vi "http XML send receive.vi"(4 "error in (no error)":errorcluster, 5 "IP-Adresse (localhost)":string="127.0.0.1", 7 "XML Request":string) -> (0 "error out":errorcluster, 2 "Response Body (XML)":string, 3 "Response Header":string)   [LabVIEW 2020, in "FT-IR.lvlib" / "TOOLweb Interface.lvlib" / "TOOLweb Interface Hilfs-VIs.lvlib"]
doc: "Der als XML-Text-Message übergebene\"XML Request\" wird mit http-POST-Header an die Anwendung ToolWeb/Cmd auf dem Rechner mit der übergebenen IP-Adresse (unverbunden: localhost) gesendet. Das Protokoll ist HTTP 1.1 auf TCP/IP.\nDie Antwort von TOOLweb wird in Response Header (bis Content-Length) und Response Body (XML) aufgeteilt. \"Response Body\" ist direkt als XML-Message auswertbar."
uses:
  TOOLweb Interface Hilfs-VIs.lvlib
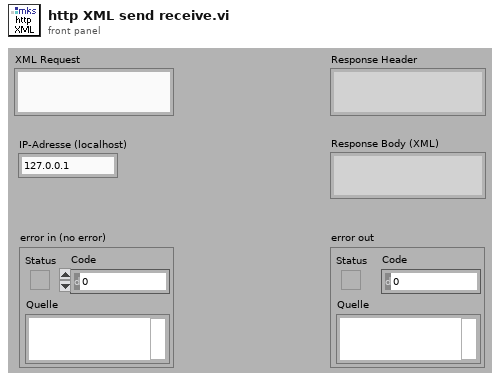
[diagram p1: front panel]
types:
  T1 = enum16{"Standard", "Buffered", "CRLF", "Immediate"}
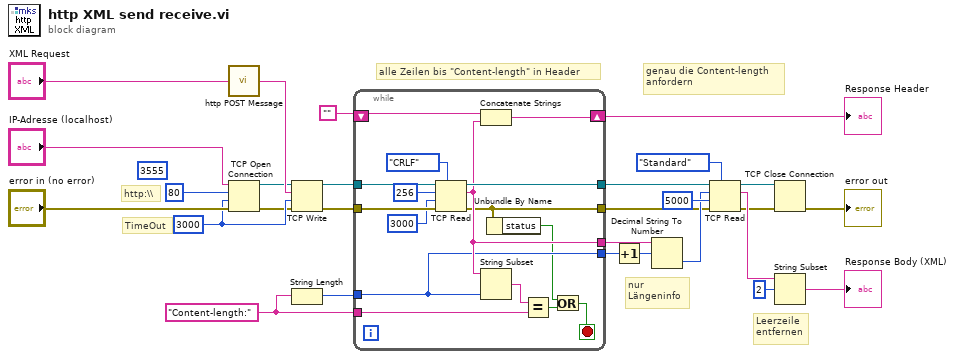
[diagram p0: block diagram]
diagram:
  (unwired) u16 3555 ("Netzwerk-Port oder -Dienst")
  w26 = "Content-length:"
  w7 = 3000 ("Timeout in ms (60000)")
  # "genau die Content-length\nanfordern"
  # "alle Zeilen bis \"Content-length\" in Header"
  # "Leerzeile\nentfernen"
  # "nur\nLängeninfo"
  # "TimeOut"
  # "http:\\\\"
  n1 = call "http POST Message.vi"("http Message Body"="XML Request") -> ("http POST Message"=w24:string)
  n2 = TCP Open Connection(address="IP-Adresse (localhost)", remote port or service name=u16 80 ("Netzwerk-Port oder -Dienst"), timeout ms (60000)=w7, error in (no error)="error in (no error)") -> (connection ID=w4:refnum<k5>, error out=w3:errorcluster)  [unwired: 1 out]
  n3 = TCP Write(connection ID=w4, data in=w24, error in (no error)=w3, 9:w7) -> (connection ID out=w5:refnum<k5>, error out=w6:errorcluster)  [unwired: 1 out]
  n4 = String Length(string=w26) -> (length=w25:i32)
  n5 = while {
    tunnel: w5 -> [w44]
    tunnel: w6 -> [w43]
    tunnel: [w32] -> w8
    tunnel: [w39] -> w10
    shift-right: [w37] -> w14
    shift-left: "" -> [w38]
    tunnel: [w35] -> w15
    tunnel: w25 -> [w33]
    tunnel: w26 -> [w34]
    tunnel: [w33] -> w28
    stop <- w29 stop-if-true
    n6 = TCP Read(connection ID=w44, bytes to read=256 ("Zu lesende Bytes"), error in (no error)=w43, 7:T1."CRLF" ("Modus (Standard)"), 9:3000 ("Timeout in ms (25000)")) -> (connection ID out=w39:refnum<k5>, data out=w35:string, error out=w32:errorcluster)
    n7 = Concatenate Strings(w38, w35) -> (w37:string)
    n8 = String Subset(string=w35, length (rest)=w33) -> (substring=w36:string)  [unwired: 1 out]
    n9 = Unbundle By Name(w32) -> ("status"=w30:bool)
    n10 = Equal?(x=w36, y=w34) -> (x = y?=w31:bool)
    n11 = Or(x=w30, y=w31) -> (x .or. y?=w29:bool)
  }
  "Response Header" <- w14
  n12 = Increment(x=w28) -> (x+1=w27:i32)
  n13 = Decimal String To Number(string=w15, offset=w27) -> (number=w16:i32)  [unwired: 2 out]
  n14 = TCP Read(connection ID=w10, bytes to read=w16, error in (no error)=w8, 7:T1."Standard" ("Modus (Standard)"), 9:5000 ("Timeout in ms (25000)")) -> (connection ID out=w11:refnum<k5>, data out=w18:string, error out=w9:errorcluster)
  n15 = TCP Close Connection(connection ID=w11, error in (no error)=w9) -> (error out=→"error out":errorcluster)  [unwired: 2 out]
  n16 = String Subset(string=w18, offset (0)=2 ("Offset (0)")) -> (substring=→"Response Body (XML)":string)  [unwired: 1 out]
